vi "Send SUBSCRIBE.vi"(8 "error in":errorcluster, 9 "Subscription Request":T8, 10 "Message Loop Data (in)":T1, 11 "WAMP Client in":refnum<class "WAMP Client.lvclass">) -> (0 "error out":errorcluster, 2 "Message Loop Data (out)":T1, 3 "WAMP Client out":refnum<class "WAMP Client.lvclass">)   [LabVIEW 2020, in "wamplv.lvlib" / "WAMP Client.lvclass"]
uses:
  WAMP Client.lvclass
  WAMP Client.lvclass/WAMP Client.ctl
  TypeDef/Subscribe Result.ctl
  TypeDef/SUBSCRIBE Request Data.ctl
  TypeDef/EVENT payload.ctl
  API/TypeDefs/WAMP error.ctl
  TypeDef/Success or error.ctl
  TypeDef/REGISTER Request Data.ctl
  TypeDef/PUBLISH Request Data.ctl
  TypeDef/Publish Requests Map.ctl
  TypeDef/Endpoint Data.ctl
  TypeDef/CALL Request Map.ctl
  TypeDef/SUBSCRIBE Requests Map.ctl
  TypeDef/Message Loop Data.ctl
  TypeDef/Subscription Details.ctl
  TypeDef/Subscriptions Map.ctl
  TypeDef/UNSUBSCRIBE Result.ctl
  TypeDef/UNSUBSCRIBE Request Data.ctl
  TypeDef/Unsubscribe Requests Map.ctl
  API/TypeDefs/Combined error.ctl
  TypeDef/Unregister request.ctl
  TypeDef/Unregister requests map.ctl
  TypeDef/PUBLISH result.ctl
  Private/Requests/ICallRequest/ICallRequest.lvclass
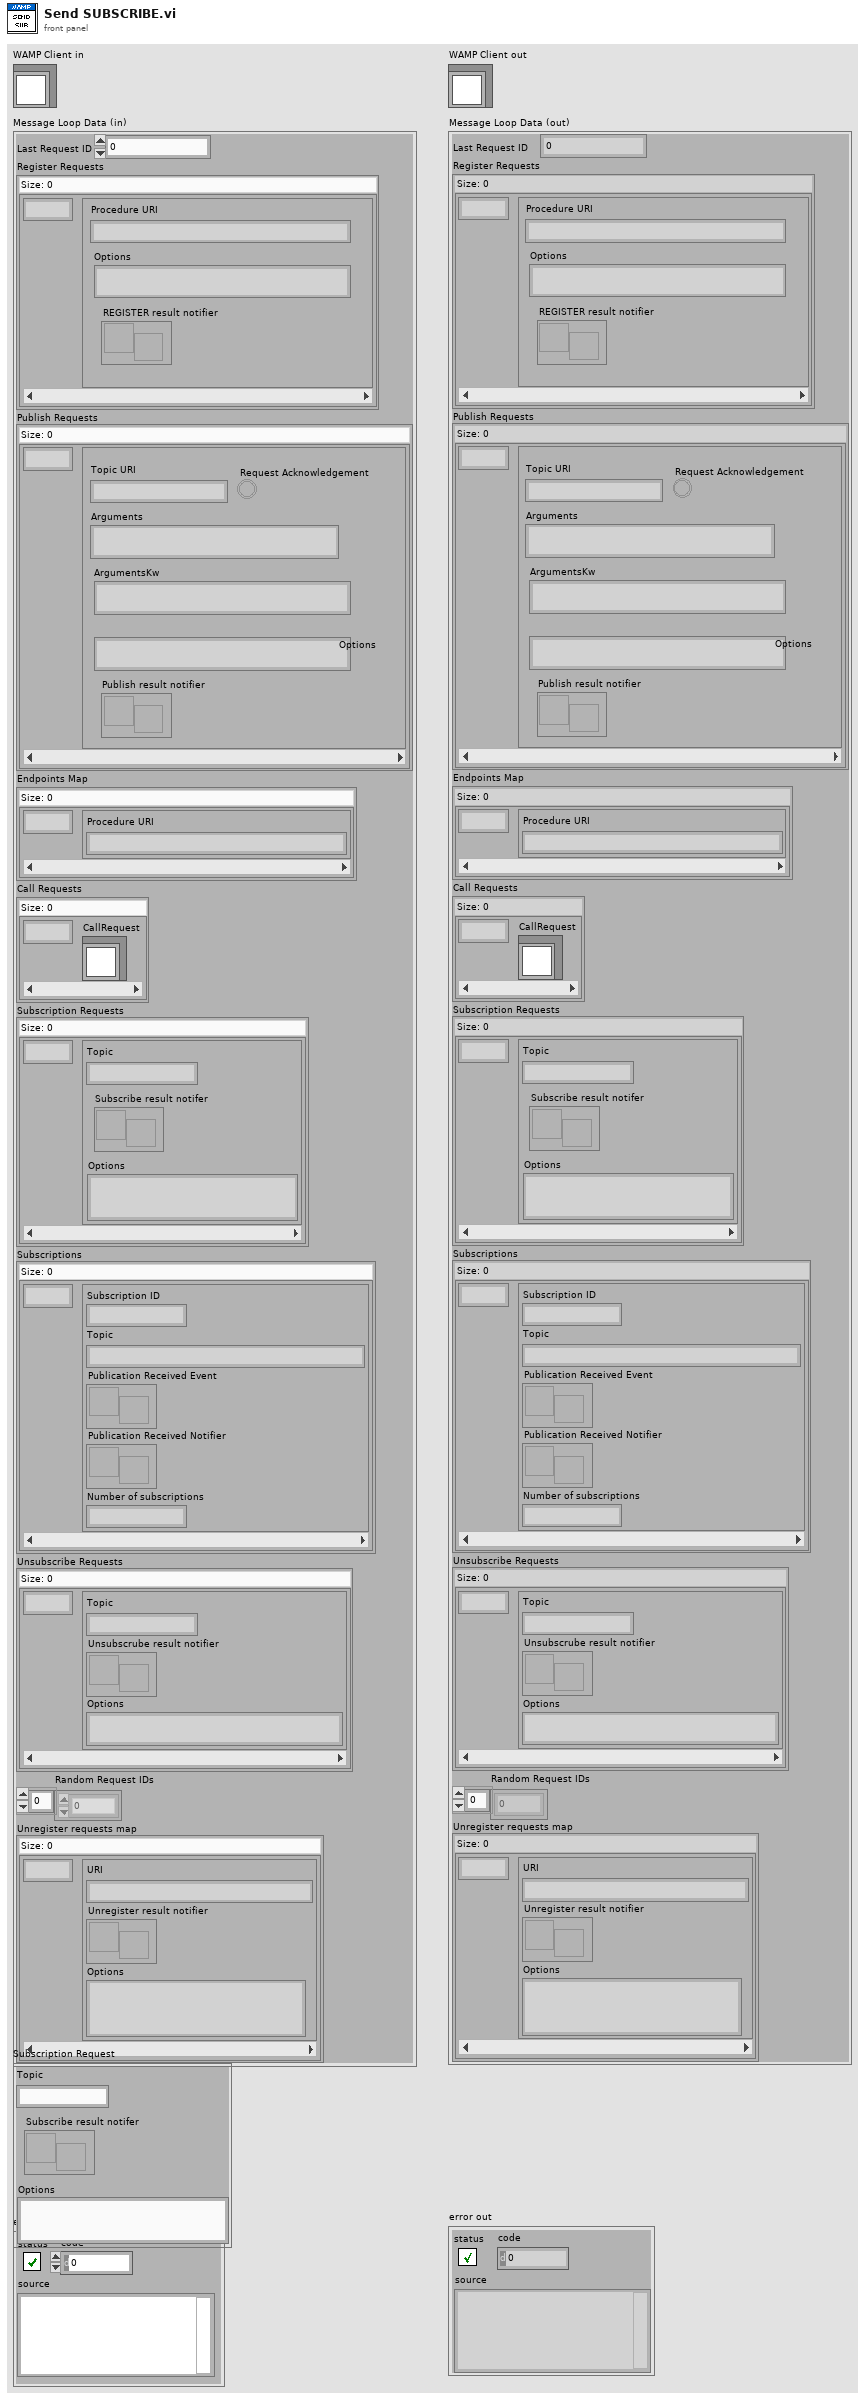
[diagram p1: front panel]
types:
  T1 = typedef "wamplv.lvlib/WAMP Client.lvclass/Message Loop Data.ctl" = cluster{"Last Request ID":u64, "Register Requests":map{u64, T2}, "Publish Requests":T3, "Endpoints Map":map{u64, T5}, "Call Requests":T6, "Subscription Requests":T7, "Subscriptions":T9, "Unsubscribe Requests":T11, "Random Request IDs":u64[], "Unregister requests map":T13}
  T2 = typedef "wamplv.lvlib/WAMP Client.lvclass/REGISTER Request Data.ctl" = cluster{"Procedure URI":string, "Options":string, "REGISTER result notifier":refnum<notifier>}
  T3 = typedef "wamplv.lvlib/WAMP Client.lvclass/Publish Requests Map.ctl" = map{u64, T4}
  T4 = typedef "wamplv.lvlib/WAMP Client.lvclass/PUBLISH Request Data.ctl" = cluster{"Topic URI":string, "Arguments":string, "ArgumentsKw":string, "Request Acknowledgement":bool, "Options":string, "Publish result notifier":refnum<notifier>}
  T5 = typedef "wamplv.lvlib/WAMP Client.lvclass/Endpoint Data.ctl" = cluster{"Procedure URI":string}
  T6 = typedef "wamplv.lvlib/WAMP Client.lvclass/CALL Request Map.ctl" = map{u64, refnum<class "ICallRequest.lvclass">}
  T7 = typedef "wamplv.lvlib/WAMP Client.lvclass/SUBSCRIBE Requests Map.ctl" = map{u64, T8}
  T8 = typedef "wamplv.lvlib/WAMP Client.lvclass/SUBSCRIBE Request Data.ctl" = cluster{"Topic":string, "Subscribe result notifer":refnum<notifier>, "Options":string}
  T9 = typedef "wamplv.lvlib/WAMP Client.lvclass/Subscriptions Map.ctl" = map{u64, T10}
  T10 = typedef "wamplv.lvlib/WAMP Client.lvclass/Subscription Details.ctl" = cluster{"Subscription ID":u64, "Topic":string, "Publication Received Event":refnum<user-event>, "Publication Received Notifier":refnum<notifier>, "Number of subscriptions":u64}
  T11 = typedef "wamplv.lvlib/WAMP Client.lvclass/Unsubscribe Requests Map.ctl" = map{u64, T12}
  T12 = typedef "wamplv.lvlib/WAMP Client.lvclass/UNSUBSCRIBE Request Data.ctl" = cluster{"Topic":string, "Unsubscrube result notifier":refnum<notifier>, "Options":string}
  T13 = typedef "wamplv.lvlib/WAMP Client.lvclass/Unregister requests map.ctl" = map{u64, T14}
  T14 = typedef "wamplv.lvlib/WAMP Client.lvclass/Unregister request.ctl" = cluster{"URI":string, "Unregister result notifier":refnum<notifier>, "Options":string}
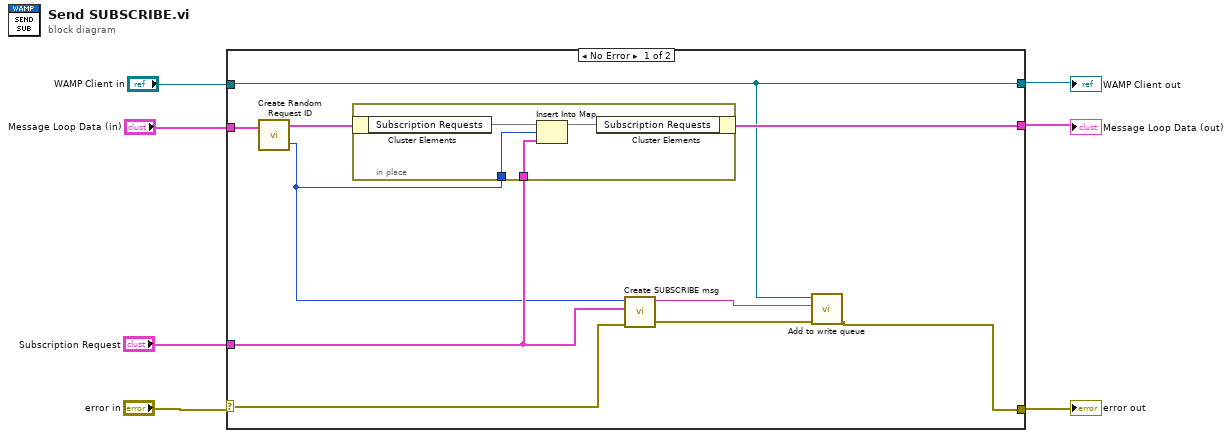
[diagram p0: block diagram]
diagram:
  n1 = case shown="No Error" "error in" {
    selector: "error in" -> [w16 w24]
    tunnel: [w8 w24] -> w6
    tunnel: [w11 w23] -> w4
    tunnel: "WAMP Client in" -> [w11 w23]
    tunnel: "Subscription Request" -> [w17 _]
    tunnel: "Message Loop Data (in)" -> [w15 w22]
    tunnel: [w12 w22] -> w1
    frame No Error {
      n2 = call "Create Random Request ID.vi"("Message Loop Shift Register Data (in)"=w15) -> ("Generated Request ID"=w14:u64, "Message Loop Shift Register Data (out)"=w13:T1)  [unwired: 1 in]
      n3 = in-place "In Place Element Structure" {
        in-place-border: w17 -> [w21]
        in-place-border: w14 -> [w20]
        n4 = in-place-cluster #1(w13) -> ("Subscription Requests"=w19:T7)
        n5 = Insert Into Map(map in=w19, key=w20, value=w21) -> (map out=w18:T7)  [unwired: 2 out]
        n6 = in-place-cluster #1("Subscription Requests"=w18) -> (w12:T1)
      }
      n7 = call "Create SUBSCRIBE msg.vi"("error in (no error)"=w16, "Subscription Request"=w17, "Request ID"=w14) -> ("error out"=w9:errorcluster, "WAMP Message"=w10:string)  [unwired: 7 in]
      n8 = call "Add to write queue.vi"("error in (no error)"=w9, "Write item"=w10, "WAMP Client in"=w11) -> ("error out"=w8:errorcluster)  [unwired: 8 in]
    }
    frame Error {
    }
  }
  "error out" <- w6
  "WAMP Client out" <- w4
  "Message Loop Data (out)" <- w1
